vi "Test CMT.vi"() -> ()   [LabVIEW 2020, in "VNA-CMT S2 S4.lvclass"]
uses:
  VNA-CMT S2 S4.lvclass
  Controls/Sparameter cluster.ctl
  C:/Sandbox/RF Bench/Source Code/WiSpry Test Framework/Instruments/Instrument.lvclass
  Instrument.lvclass/Instrument.ctl
  Instrument.lvclass
  Vector Network Analyzer.lvclass
panel:
  out "S parameters":T1[](array[typedef])
  in  "Sparameters (string)":string[](array[string])=["S11", "S12", "S21", "S22"]
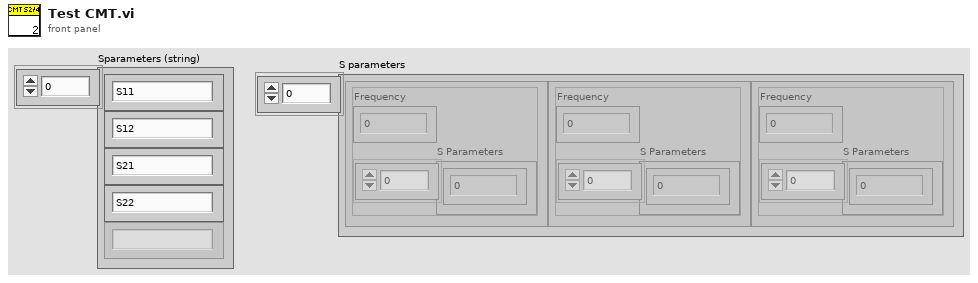
[diagram p1: front panel]
types:
  T1 = typedef "Vector Network Analyzer.lvclass/Sparameter cluster.ctl" = cluster{"Frequency":dbl, "S Parameters":cdb[]}
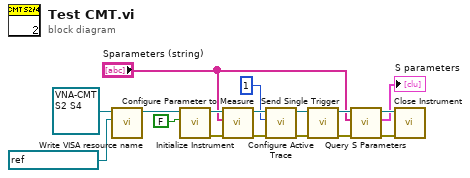
[diagram p0: block diagram]
diagram:
  n1 = call "Write VISA resource name.vi"("VISA resource name"=refnum<visa-resource-name> "CMT_C1409", "Instrument in"=refnum<class "VNA-CMT S2 S4.lvclass"> refnum ("VNA-CMT S2 S4.lvclass")) -> ("Instrument out"=w9:refnum<class "VNA-CMT S2 S4.lvclass">)  [unwired: 9 in]
  n2 = call-dynamic "Initialize Instrument.vi"("Reset"=FALSE, "VNA-CMT S2 S4 in"=w9) -> ("error out"=w14:errorcluster, "VNA-CMT S2 S4 out"=w13:refnum<class "VNA-CMT S2 S4.lvclass">)  [unwired: 8 in]
  n3 = call-dynamic "Configure Parameter to Measure.vi"("error in (no error)"=w14, "Sparameters (string)"="Sparameters (string)", "VNA-CMT S2 S4 in"=w13) -> ("error out"=w12:errorcluster, "VNA-CMT S2 S4 out"=w11:refnum<class "VNA-CMT S2 S4.lvclass">)  [unwired: 7 in]
  n4 = call-dynamic "Configure Active Trace.vi"("error in (no error)"=w12, "Active Trace"=u8 1, "VNA-CMT S2 S4 in"=w11) -> ("error out"=w6:errorcluster, "VNA-CMT S2 S4 out"=w7:refnum<class "VNA-CMT S2 S4.lvclass">)  [unwired: 7 in]
  n5 = call-dynamic "Send Single Trigger.vi"("error in (no error)"=w6, "VNA-CMT S2 S4 in"=w7) -> ("error out"=w8:errorcluster, "VNA-CMT S2 S4 out"=w5:refnum<class "VNA-CMT S2 S4.lvclass">)  [unwired: 8 in]
  n6 = call-dynamic "Query S Parameters.vi"("error in (no error)"=w8, "Sparameters (string)"="Sparameters (string)", "VNA-CMT S2 S4 in"=w5) -> ("error out"=w3:errorcluster, "S parameters"=→"S parameters":T1[], "VNA-CMT S2 S4 out"=w4:refnum<class "VNA-CMT S2 S4.lvclass">)  [unwired: 6 in]
  n7 = call-dynamic "Close Instrument.vi"("error in (no error)"=w3, "Instrument in"=w4) -> ()  [unwired: 8 in, 2 out]
